vi "Add.vi"() -> ()   [LabVIEW 2017]
panel:
  out "x+y":dbl
  in  "y":dbl
  in  "x":dbl
  # "added file"
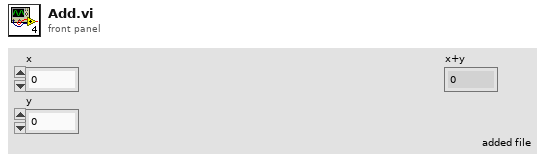
[diagram p1: front panel]
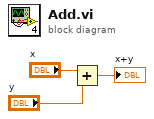
[diagram p0: block diagram]
diagram:
  n1 = Add(x="x", y="y") -> (x+y=→"x+y":dbl)
